vi "ID解析.vi"(11 "ID":i32 format="%x") -> (0 "SA(4)":i32 format="%x", 1 "PS(3)":i32 format="%x", 2 "PF(2)":i32 format="%x", 3 "PDU(1)":i32 format="%x", 5 "前三组合":string)   [LabVIEW 2013]
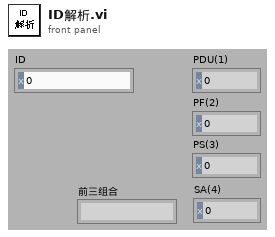
[diagram p1: front panel]
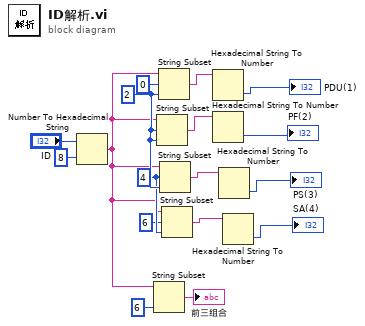
[diagram p0: block diagram]
diagram:
  w14 = 4 ("偏移量(0)")
  w15 = 2 ("长度（剩余）")
  n1 = Number To Hexadecimal String(1:i16 8 ("宽度(-)"), 2:"ID") -> (0:w3:string)
  n2 = String Subset(string=w3, length (rest)=6 ("长度（剩余）")) -> (substring=→"前三组合":string)  [unwired: 1 out]
  n3 = String Subset(string=w3, offset (0)=w15, length (rest)=w15) -> (substring=w10:string)
  n4 = String Subset(string=w3, offset (0)=0 ("偏移量(0)"), length (rest)=w15) -> (substring=w12:string)
  n5 = String Subset(string=w3, offset (0)=w14, length (rest)=w15) -> (substring=w8:string)
  n6 = String Subset(string=w3, offset (0)=6 ("偏移量(0)"), length (rest)=w14) -> (substring=w6:string)
  n7 = Hexadecimal String To Number(string=w12) -> (number=→"PDU(1)":u32)  [unwired: 3 out]
  n8 = Hexadecimal String To Number(string=w10) -> (number=→"PF(2)":u32)  [unwired: 3 out]
  n9 = Hexadecimal String To Number(string=w8) -> (number=→"PS(3)":u32)  [unwired: 3 out]
  n10 = Hexadecimal String To Number(string=w6) -> (number=→"SA(4)":u32)  [unwired: 3 out]
